vi "Select Specifc Bit Values.vi"(4 "#ofBits":u8=1 min=1 max=8, 6 "Bit_Location(LSB)":u8 max=7, 11 "Converted Data":T1 {"Register" format="%.0x"; "Slave Address" max=15 format="%.0x"}) -> (3 "Bits":u8=184)   [LabVIEW 2013]
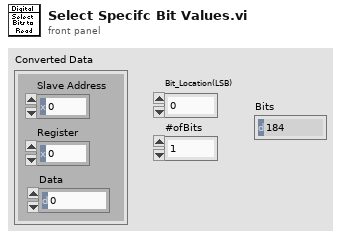
[diagram p1: front panel]
types:
  T1 = cluster{"Slave Address":u8, "Register":u8, "Data":u8}
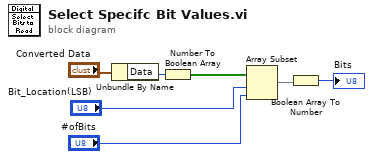
[diagram p0: block diagram]
diagram:
  n1 = Unbundle By Name("Converted Data") -> ("Data"=w6:u8)
  n2 = Number To Boolean Array(number=w6) -> (Boolean array=w2:bool[])
  n3 = Array Subset(array=w2, index="Bit_Location(LSB)", length="#ofBits") -> (w1:bool[])
  n4 = Boolean Array To Number(Boolean array=w1) -> (number=→"Bits":u32)
